vi "Scatter plot cursors.vi"(0 "Peaks":refnum<vi>, 1 "autoscale":bool, 2 "center cursors":bool) -> ()   [LabVIEW 2009]
uses:
  <vilib>/Utility/miscctls.llb/LVCursorListTypeDef.ctl
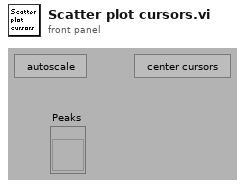
[diagram p1: front panel]
types:
  T1 = typedef "LVCursorListTypeDef.ctl" = cluster{"Name":string, "Color":u32, "Style":u8, "Point Style":u8, "Name Visible":bool, "Allow Drag":bool, "Cursor Mode":u32, "Plot":i32, "Index":i32, "Position":cluster{"X":dbl, "Y":dbl}, "X Scale":u32, "Y Scale":u32, "Watch Plots":i32[], "Watch All Plots":bool, "Plot Area":i32, "Label Offset":cluster{"X":dbl, "Y":dbl}}[]
  T2 = cluster{"Name":string, "Color":u32, "Style":u8, "Point Style":u8, "Name Visible":bool, "Allow Drag":bool, "Cursor Mode":u32, "Plot":i32, "Index":i32, "Position":cluster{"X":dbl, "Y":dbl}, "X Scale":u32, "Y Scale":u32, "Watch Plots":i32[], "Watch All Plots":bool, "Plot Area":i32, "Label Offset":cluster{"X":dbl, "Y":dbl}}
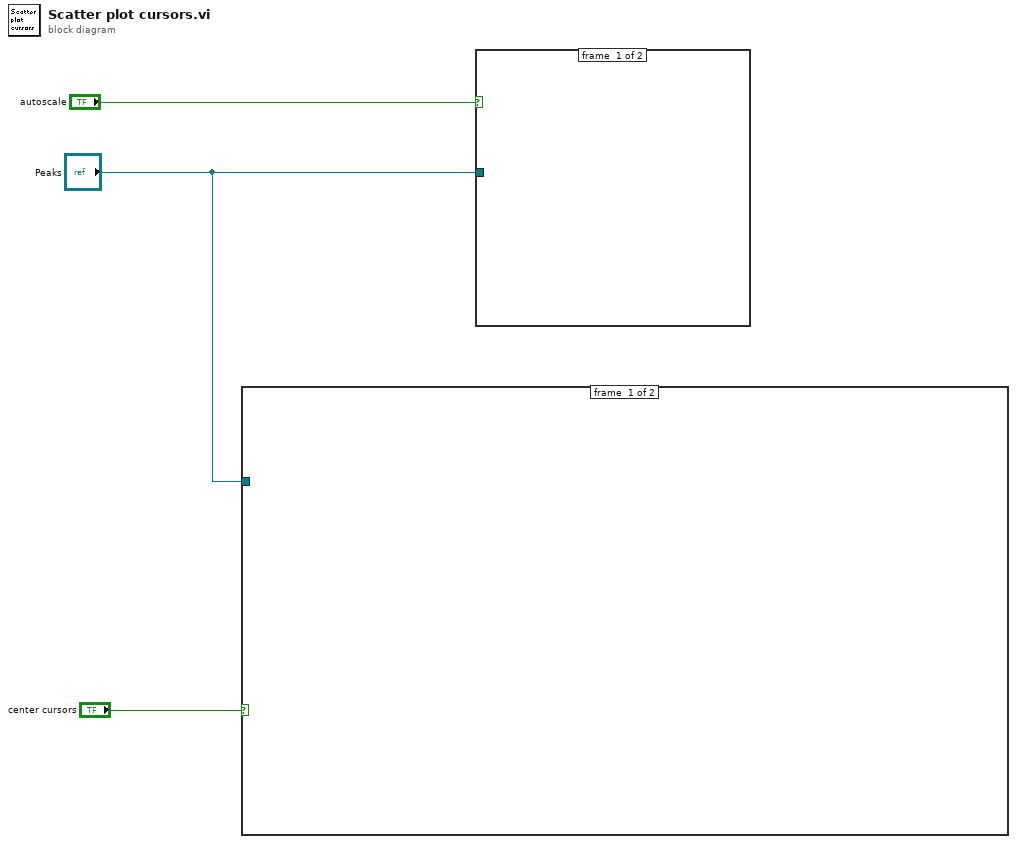
[diagram p0: block diagram]
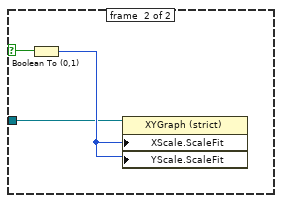
[diagram p2: hidden frame]
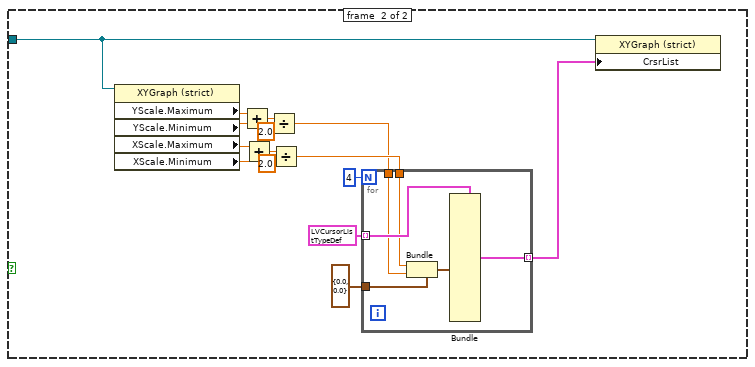
[diagram p3: hidden frame]
diagram:
  n1 = case shown="True" "center cursors" {
    tunnel: "Peaks" -> [_ w4]
    frame #0 {
    }
    frame #1 {
      n2 = property on="Property Node" class="XYGraph (strict)"(reference=w4) -> ("YScale.Maximum"=w11:dbl, "YScale.Minimum"=w12:dbl, "XScale.Maximum"=w18:dbl, "XScale.Minimum"=w17:dbl)  [unwired: 1 in, 2 out]
      n3 = Add(x=w11, y=w12) -> (x+y=w13:dbl)
      n4 = Add(x=w18, y=w17) -> (x+y=w16:dbl)
      n5 = Divide(x=w13, y=2.0) -> (x/y=w5:dbl)
      n6 = Divide(x=w16, y=2.0) -> (x/y=w6:dbl)
      n7 = for {
        N: 4 -> [_]
        tunnel: T1 [{"Name"="0", "Color"=16713728, "Style"=0, "Point Style"=13, "Name Visible"=FALSE, "Allow Drag"=TRUE, "Cursor Mode"=0, "Plot"=0, "Index"=0, "Position"={"X"=0.0104, "Y"=0.0}, "X Scale"=0, "Y Scale"=0, "Watch Plots"=[], "Watch All Plots"=FALSE, "Plot Area"=0, "Label Offset"={"X"=-2.7779731345449823e-06, "Y"=0.0002945665445665416}}, {"Name"="1", "Color"=16773698, "Style"=0, "Point Style"=13, "Name Visible"=FALSE, "Allow Drag"=TRUE, "Cursor Mode"=0, "Plot"=0, "Index"=0, "Position"={"X"=0.005296610169491526, "Y"=0.0010952380952380953}, "X Scale"=0, "Y Scale"=0, "Watch Plots"=[], "Watch All Plots"=FALSE, "Plot Area"=0, "Label Offset"={"X"=2.1450172304621207e-06, "Y"=0.0003021978021977979}}, {"Name"="2", "Color"=3473194, "Style"=0, "Point Style"=13, "Name Visible"=FALSE, "Allow Drag"=TRUE, "Cursor Mode"=0, "Plot"=0, "Index"=0, "Position"={"X"=0.005127118644067797, "Y"=0.008095238095238096}, "X Scale"=0, "Y Scale"=0, "Watch Plots"=[], "Watch All Plots"=FALSE, "Plot Area"=0, "Label Offset"={"X"=-2.6373162669715913e-06, "Y"=0.0003021978021978001}}, {"Name"="3", "Color"=1187327, "Style"=0, "Point Style"=13, "Name Visible"=FALSE, "Allow Drag"=TRUE, "Cursor Mode"=0, "Plot"=0, "Index"=0, "Position"={"X"=0.009279661016949154, "Y"=0.0037606837606837607}, "X Scale"=0, "Y Scale"=0, "Watch Plots"=[], "Watch All Plots"=FALSE, "Plot Area"=0, "Label Offset"={"X"=2.4966593993938635e-06, "Y"=0.000299145299145296}}] ("Cursor List") -> [w24] mode=indexing
        tunnel: cluster{"X":dbl, "Y":dbl} {"X"=0.0, "Y"=0.0} ("Position") -> [w23]
        tunnel: w5 -> [w21]
        tunnel: w6 -> [w20]
        tunnel: [w19] -> w7 mode=indexing
        n8 = Bundle(cluster=w23, "X"=w20, "Y"=w21) -> (w22:cluster{"X":dbl, "Y":dbl})
        n9 = Bundle(cluster=w24, "Position"=w22) -> (w19:T2)  [unwired: 15 in]
      }
      n10 = property on="Property Node" class="XYGraph (strict)"(reference=w4, "CrsrList"=w7) -> ()  [unwired: 1 in, 2 out]
    }
  }
  n11 = case shown="True" "autoscale" {
    selector: "autoscale" -> [_ w26]
    tunnel: "Peaks" -> [_ w25]
    frame #0 {
    }
    frame #1 {
      n12 = Boolean To (0,1)(Boolean=w26) -> (0, 1=w27:i16)
      n13 = property on="Property Node" class="XYGraph (strict)"(reference=w25, "XScale.ScaleFit"=w27, "YScale.ScaleFit"=w27) -> ()  [unwired: 1 in, 2 out]
    }
  }
